vi "oldAllyTeamToOOAllyTeam.vi"(8 "error in (no error)":errorcluster, 10 "our_robots":T1[](array[typedef]) {"height" format="%+4.3f"; "pixel_y" format="%+4.3f"; "pixel_x" format="%+4.3f"; "orientation" format="%+4.3f"; "y" format="%+4.3f"; "confidence" format="%4.3f"; "x" format="%+4.3f"}, 11 "Game in":refnum<class "Game.lvclass">) -> (0 "error out":errorcluster, 3 "Game out":refnum<class "Game.lvclass">)   [LabVIEW 2018]
uses:
  Ally_class/Ally.lvclass
  Robot_class/Robot.lvclass
  Game.lvclass
  <vilib>/Analysis/Matrix/Datatypes/RealMatrix.ctl
  <vilib>/Analysis/Matrix/NI_Matrix.lvlib
  Vision_class/Old vision/Controls/SSL Detection Robot.ctl
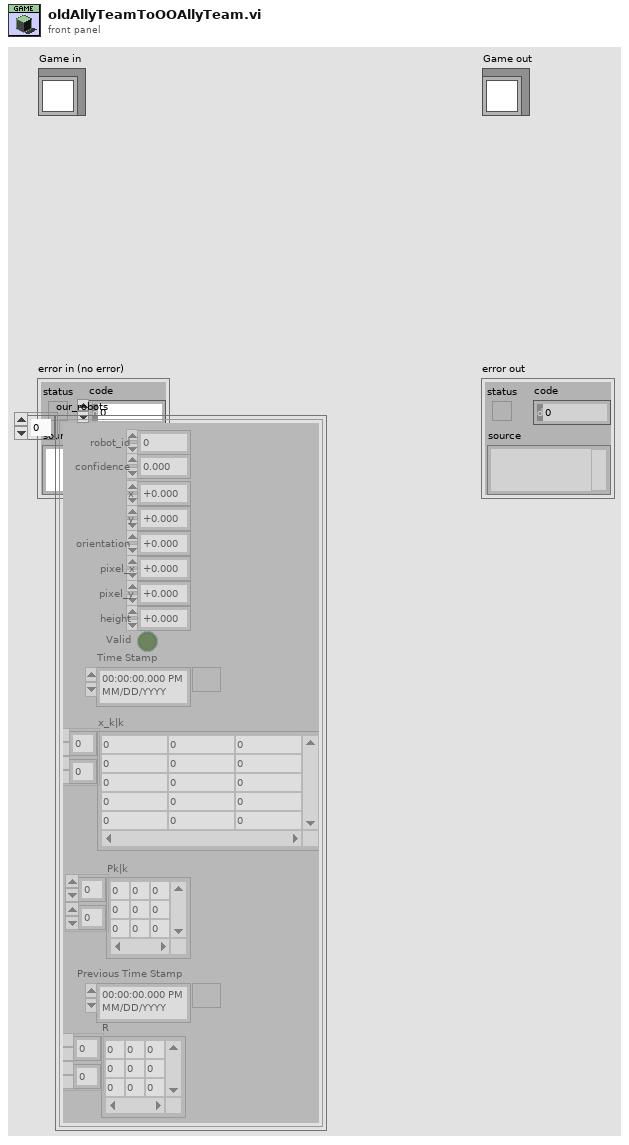
[diagram p1: front panel]
types:
  T1 = typedef "SSL Detection Robot.ctl" = cluster{"x":sgl, "robot_id":u32, "confidence":sgl, "y":sgl, "orientation":sgl, "pixel_x":sgl, "pixel_y":sgl, "height":sgl, "Valid":bool, "Time Stamp":timestamp, "x_k|k":T2, "Pk|k":T2, "Previous Time Stamp":timestamp, "R":T2}
  T2 = typedef "NI_Matrix.lvlib/RealMatrix.ctl" = dbl[][]
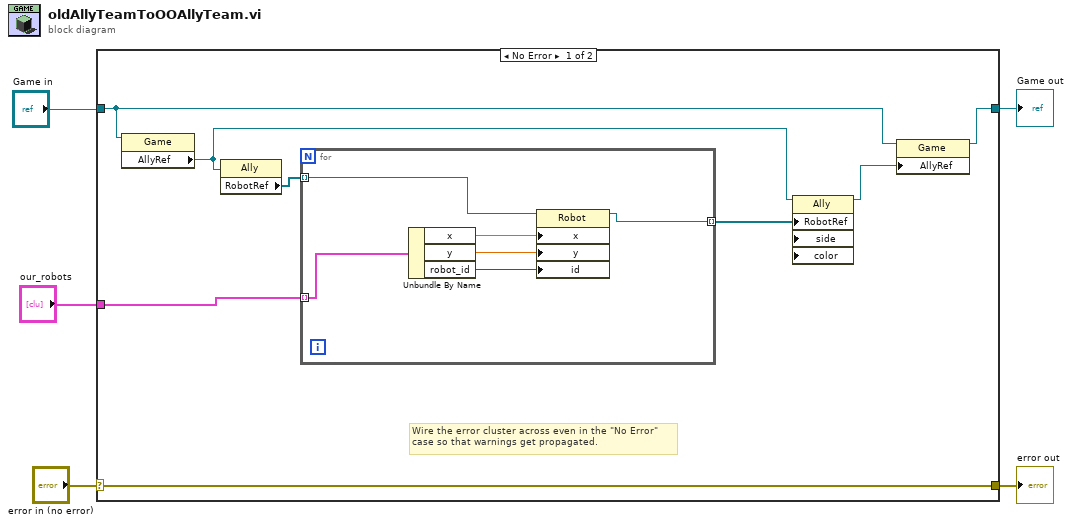
[diagram p0: block diagram]
diagram:
  n1 = case shown="No Error" "error in (no error)" {
    selector: "error in (no error)" -> [w13 w21]
    tunnel: [w13 w21] -> w4
    tunnel: [w8 w20] -> w2
    tunnel: "Game in" -> [w7 w20]
    tunnel: "our_robots" -> [w12 _]
    frame No Error {
      # "Wire the error cluster across even in the \"No Error\"\ncase so that warnings get propagated."
      n2 = property class="Game"(reference=w7) -> ("AllyRef"=w6:refnum<class "Ally.lvclass">)  [unwired: 1 in, 2 out]
      n3 = property class="Ally"(reference=w6) -> ("RobotRef"=w11:refnum<class "Robot.lvclass">[])  [unwired: 1 in, 2 out]
      n4 = for {
        tunnel: w12 -> [w19] mode=indexing
        tunnel: w11 -> [w18] mode=indexing
        tunnel: [w14] -> w10 mode=indexing
        n5 = Unbundle By Name(w19) -> ("x"=w17:sgl, "y"=w16:sgl, "robot_id"=w15:u32)
        n6 = property class="Robot"(reference=w18, "x"=w17, "y"=w16, "id"=w15) -> (reference out=w14:refnum<class "Robot.lvclass">)  [unwired: 1 in, 1 out]
      }
      n7 = property class="Ally" props=["RobotRef", "side", "color"](reference=w6, "RobotRef"=w10) -> (reference out=w9:refnum<class "Ally.lvclass">)  [unwired: 3 in, 1 out]
      n8 = property class="Game"(reference=w7, "AllyRef"=w9) -> (reference out=w8:refnum<class "Game.lvclass">)  [unwired: 1 in, 1 out]
    }
    frame Error {
    }
  }
  "error out" <- w4
  "Game out" <- w2
